vi "route.vi"() -> ()   [LabVIEW 2014]
uses:
  <vilib>/Utility/sysdir.llb/System Directory Type.ctl
  <vilib>/Utility/config.llb/Read Key (String).vi
  <vilib>/Utility/config.llb/Write Key (String).vi
  subVI/version.vi
  <vilib>/Utility/config.llb/Read Key (Path).vi
  <vilib>/Utility/config.llb/Write Key (Path).vi
  subVI/departure.vi
  subVI/Destination.vi
  <vilib>/Utility/file.llb/Write To Spreadsheet File (string).vi
  <vilib>/httpClient/LabVIEWHTTPClient.lvlib
  <vilib>/Utility/config.llb/NI_LVConfig.lvlib
panel:
  in  "ATC":bool
  out "활주로":string[](array[string])
  out "fms":string
  out "time/시간":dbl
  in  "도움말":bool
  in  "피드백":bool
  in  "저장 경로":path
  out "Distance":string="0"
  in  "찾기":bool
  in  "?":bool
  in  "?":bool
  out "x fmc 플랜":string
  out "FMS 플랜":string
  in  "Destination":string
  in  "departure":string
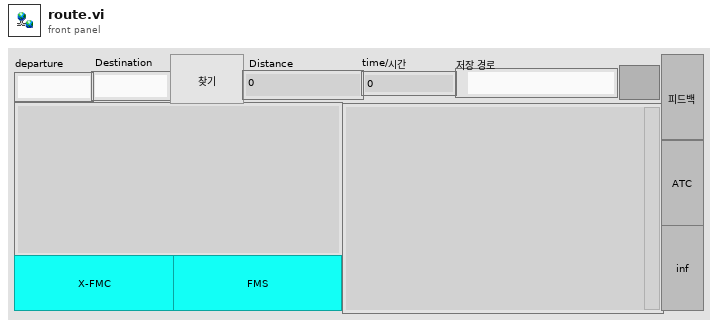
[diagram p1: front panel]
types:
  T1 = enum16{"open", "replace", "create", "open or create", "replace or create", "replace or create with confirmation"}
  T2 = typedef "NI_LVConfig.lvlib/Config Data RefNum.ctl" = refnum<k1>
  T3 = typedef "System Directory Type.ctl" = i32
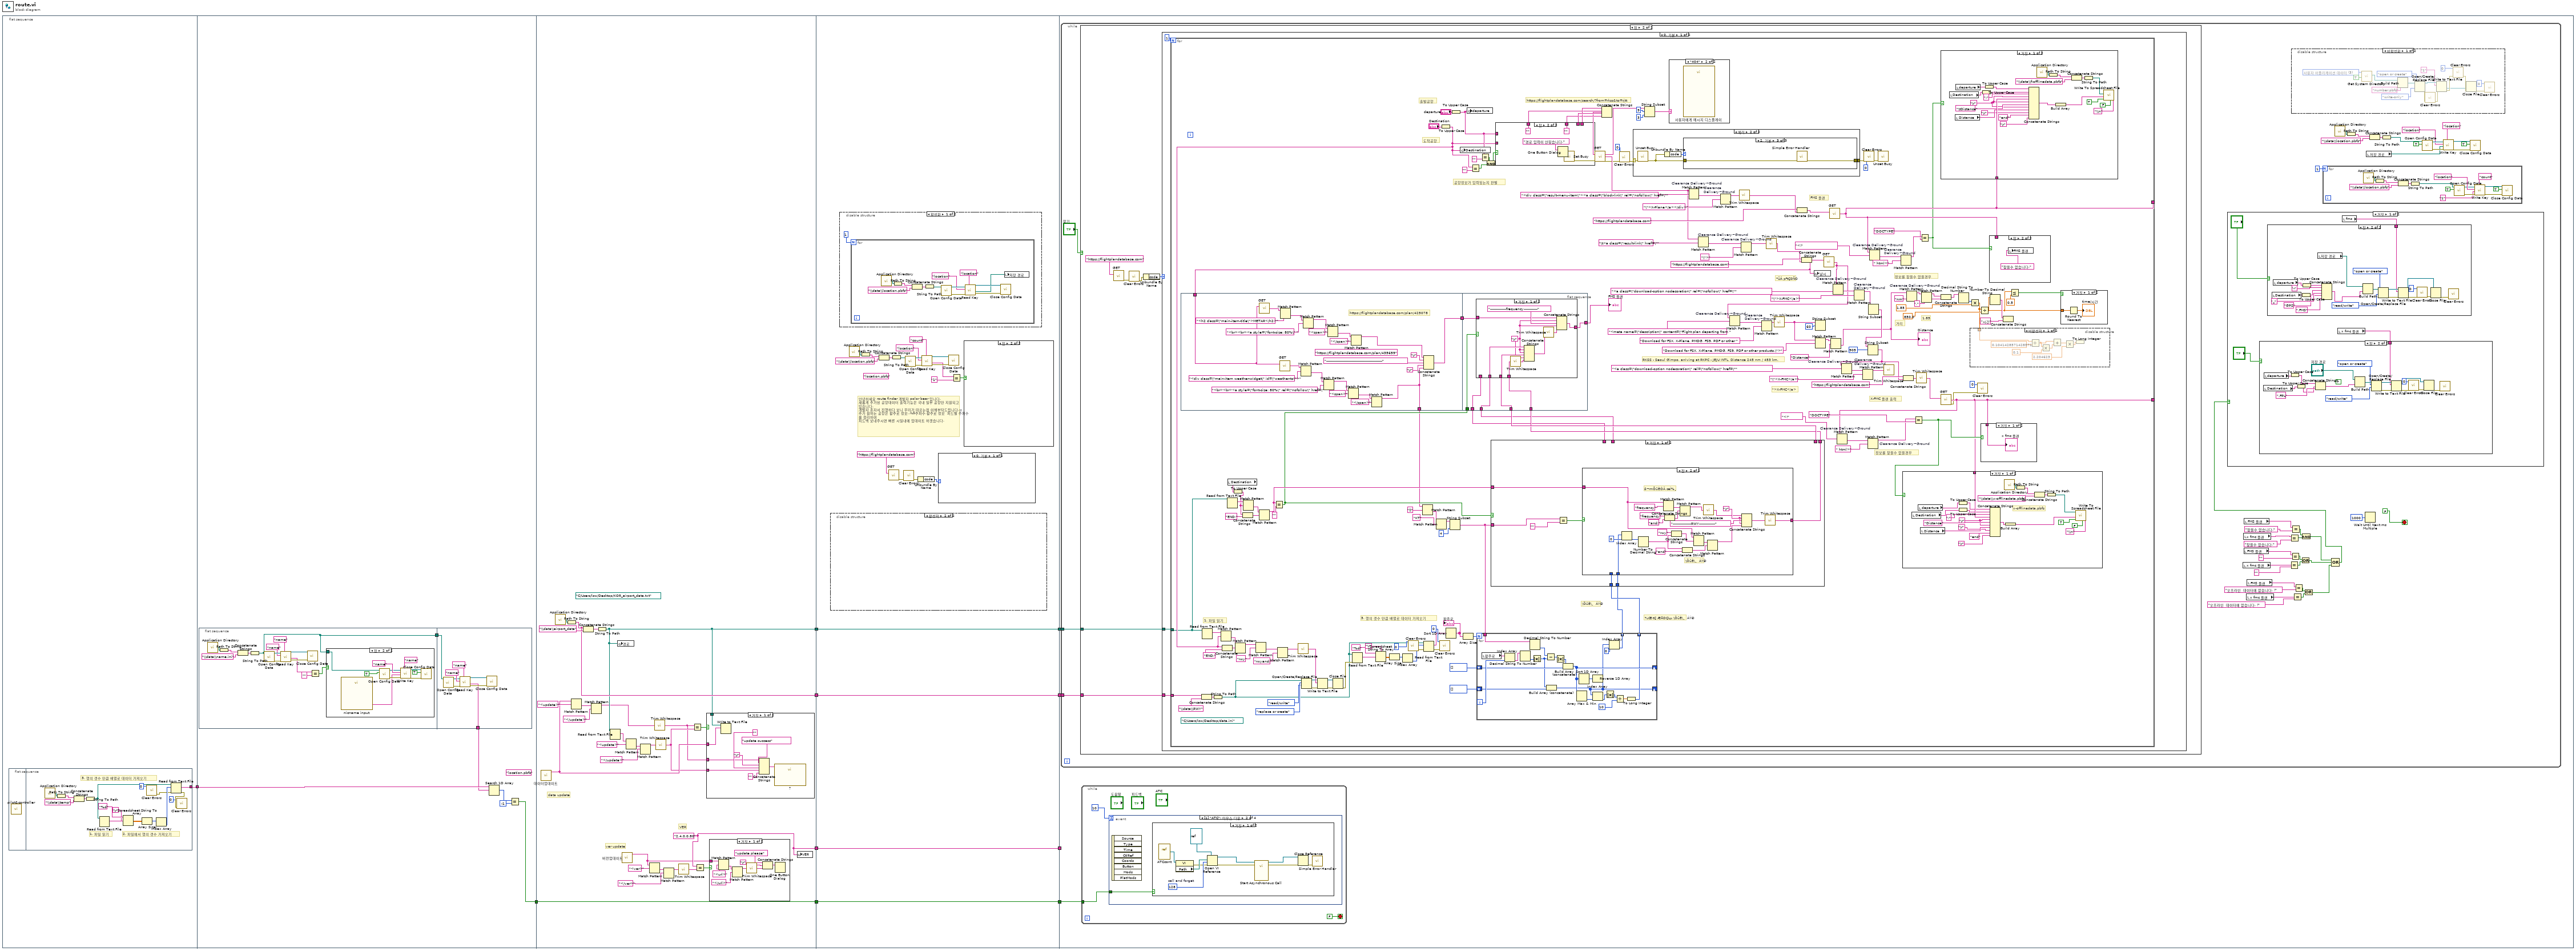
[diagram p0: block diagram]
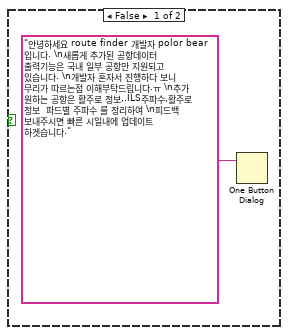
[diagram p5: hidden frame]
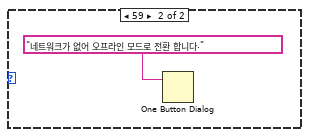
[diagram p6: hidden frame]
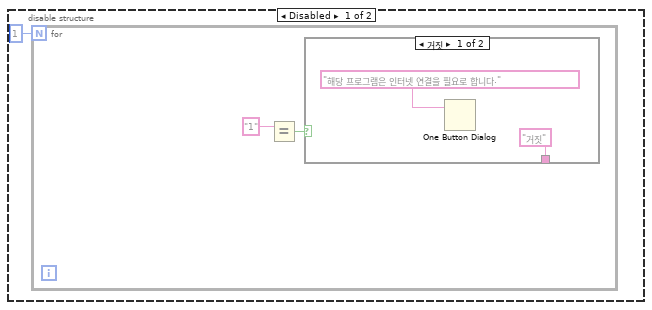
[diagram p7: hidden frame]
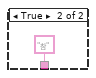
[diagram p8: hidden frame]
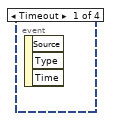
[diagram p10: hidden frame]
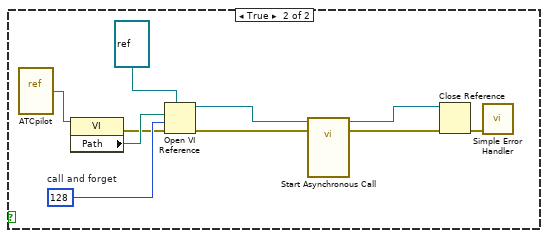
[diagram p11: hidden frame]
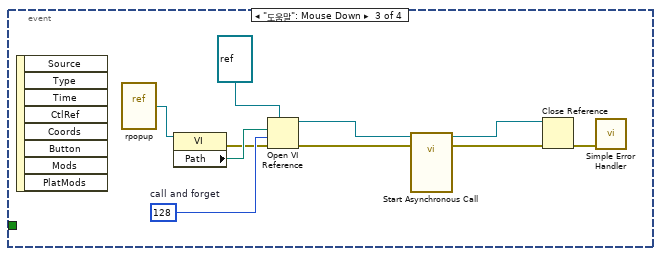
[diagram p12: hidden frame]
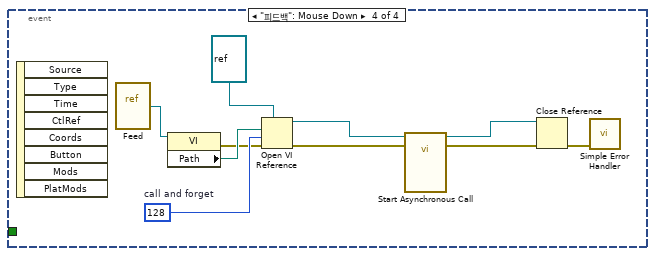
[diagram p13: hidden frame]
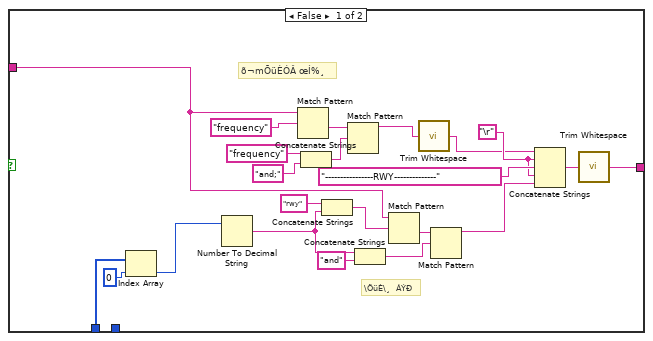
[diagram p15: hidden frame]
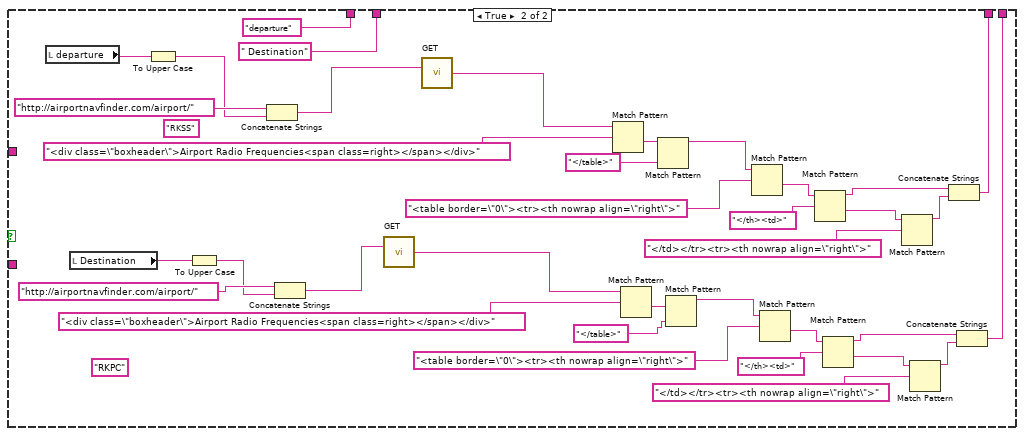
[diagram p16: hidden frame]
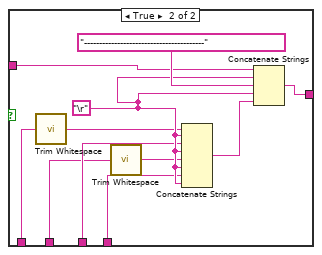
[diagram p17: hidden frame]
diagram:
  n1 = flat-sequence {
    tunnel: [w11] -> w4
    tunnel: w4 -> [w33]
    tunnel: [w31] -> w3
    tunnel: [w89] -> w8
    tunnel: [w90] -> w7
    tunnel: [w69] -> w6
    tunnel: w3 -> [w66]
    tunnel: [w66] -> w2
    tunnel: [w113] -> w10
    tunnel: [w114] -> w9
    tunnel: w8 -> [w113]
    tunnel: w7 -> [w114]
    tunnel: w6 -> [w112]
    tunnel: [w112] -> w5
    tunnel: w2 -> [w111]
    tunnel: [w111] -> w1
    tunnel: w10 -> [w156]
    tunnel: w9 -> [w155]
    tunnel: w5 -> [_]
    tunnel: w1 -> [w154]
    frame #0 {
      n2 = flat-sequence {
        tunnel: [w16] -> w11
        frame #0 {
          n3 = call "pilot&controller.vi"() -> ()  [unwired: 11 in, 1 out]
        }
        frame #1 {
          # "3. 행의 갯수 만큼 배열로 데이터 가져오기"
          # "2. 파일에서 행의 갯수 가져오기"
          # "1. 파일 읽기"
          n4 = call <vilib>:"Application Directory.vi"() -> ("Application Directory"=w20:path)
          n5 = Path To String(path=w20) -> (string=w19:string)
          n6 = Concatenate Strings(w19, "\\data\\temp" ("문자열")) -> (w18:string)
          n7 = String To Path(string=w18) -> (path=w17:path)
          n8 = Read from Text File(file (use dialog)=w17) -> (text=w23:string)  [unwired: 1 in, 5 out]
          n9 = Spreadsheet String To Array(delimiter (Tab)="\r", format string="%d", spreadsheet string=w23) -> (array=w25:dbl[][])  [unwired: 1 out]
          n10 = Array Size(array=w25) -> (size(s)=w24:i32[])
          n11 = call <vilib>:"Clear Errors.vi"("specific error code to clear (0: all)"=0) -> ("error out"=w15:errorcluster)  [unwired: 5 in, 1 out]
          n12 = Index Array(array=w24) -> (element=w22:i32)  [unwired: 1 in]
          n13 = Read from Text File(file (use dialog)=w17, count=w22, error in=w15) -> (text=w16:string[], error out=w13:errorcluster)  [unwired: 3 out]
          n14 = call <vilib>:"Clear Errors.vi"("error in (no error)"=w13, "specific error code to clear (0: all)"=0) -> ()  [unwired: 4 in, 2 out]
        }
      }
    }
    frame #1 {
      (unwired) "location.pbfs" ("문자열")
      n15 = flat-sequence {
        tunnel: [w34] -> w28
        tunnel: [w59] -> w30
        tunnel: w28 -> [w58]
        frame #0 {
          n16 = call <vilib>:"Application Directory.vi"() -> ("Application Directory"=w40:path)
          n17 = Path To String(path=w40) -> (string=w38:string)
          n18 = Concatenate Strings(w38, "\\data\\name.ini" ("문자열")) -> (w39:string)
          n19 = String To Path(string=w39) -> (path=w34:path)
          n20 = call <vilib>:"Open Config Data.vi"("configuration file path"=w34) -> ("error out"=w45:errorcluster, "refnum"=w46:T2)  [unwired: 8 in, 1 out]
          n21 = call-poly <vilib>:"Read Key.vi"("section"="name", "error in (no error)"=w45, "key"="name", "refnum"=w46) -> ("error out"=w44:errorcluster, "value"=w35:string, "refnum out"=w43:T2)  [unwired: 4 in, 1 out]
          n22 = call <vilib>:"Close Config Data.vi"("error in (no error)"=w44, "refnum"=w43) -> ()  [unwired: 8 in, 2 out]
          n23 = Equal?(x=w35, y="") -> (x = y?=w36:bool)
          n24 = case shown="참" w36 {
            tunnel: w34 -> [_ w48]
            frame False {
            }
            frame True {
              n25 = call "nicname input"() -> ("nicname"=w49:string)  [unwired: 17 in, 2 out]
              n26 = call <vilib>:"Open Config Data.vi"("create file if necessary (T)"=TRUE, "configuration file path"=w48) -> ("error out"=w51:errorcluster, "refnum"=w52:T2)  [unwired: 7 in, 1 out]
              n27 = call-poly <vilib>:"Write Key.vi"("section"="name", "error in (no error)"=w51, "value"=w49, "key"="name", "refnum"=w52) -> ("error out"=w54:errorcluster, "refnum out"=w53:T2)  [unwired: 4 in, 1 out]
              n28 = call <vilib>:"Close Config Data.vi"("error in (no error)"=w54, "write file if changed (T)"=TRUE, "refnum"=w53) -> ()  [unwired: 7 in, 2 out]
            }
          }
        }
        frame #1 {
          n29 = call <vilib>:"Open Config Data.vi"("configuration file path"=w58) -> ("error out"=w62:errorcluster, "refnum"=w61:T2)  [unwired: 8 in, 1 out]
          n30 = call-poly <vilib>:"Read Key.vi"("section"="name", "error in (no error)"=w62, "key"="name", "refnum"=w61) -> ("error out"=w63:errorcluster, "value"=w59:string, "refnum out"=w64:T2)  [unwired: 4 in, 1 out]
          n31 = call <vilib>:"Close Config Data.vi"("error in (no error)"=w63, "refnum"=w64) -> ()  [unwired: 8 in, 2 out]
        }
      }
      n32 = Search 1D Array(1D array=w33, element=w30) -> (index of element=w32:i32)  [unwired: 1 in]
      n33 = Equal?(x=w32, y=-1) -> (x = y?=w31:bool)
    }
    frame #2 {
      w69 = "2.4.0.0.80"
      (unwired) path "C:/Users/lsw/Desktop/KOR_airport_data.txt" ("File Path Control")
      # "ver update"
      # "data update"
      # "VER"
      n34 = call "데이터업데이트.vi"() -> ("data"=w78:string)  [unwired: 11 in]
      n35 = call <vilib>:"Application Directory.vi"() -> ("Application Directory"=w92:path)
      n36 = Path To String(path=w92) -> (string=w90:string)
      n37 = Match Pattern(string=w78, regular expression="<update>" ("정규식")) -> (after substring=w86:string)  [unwired: 1 in, 3 out]
      n38 = Concatenate Strings(w90, "\\data\\airport_data" ("문자열")) -> (w88:string)
      n39 = Match Pattern(string=w86, regular expression="</update>" ("정규식")) -> (before substring=w80:string)  [unwired: 1 in, 3 out]
      n40 = String To Path(string=w88) -> (path=w89:path)
      n41 = Read from Text File(file (use dialog)=w89) -> (text=w81:string)  [unwired: 3 in, 3 out]
      n42 = global write "airport경로.vi" "경로"(w89) -> ()
      n43 = call "버전업데이트.vi"() -> ("data"=w67:string)  [unwired: 11 in]
      n44 = Match Pattern(string=w81, regular expression="<update>" ("정규식")) -> (after substring=w83:string)  [unwired: 1 in, 3 out]
      n45 = Match Pattern(string=w83, regular expression="</update>" ("정규식")) -> (before substring=w79:string)  [unwired: 1 in, 3 out]
      n46 = Match Pattern(string=w67, regular expression="<ver>" ("정규식")) -> (after substring=w74:string)  [unwired: 1 in, 3 out]
      n47 = call <vilib>:"Trim Whitespace.vi"("string"=w80) -> ("trimmed string"=w76:string)  [unwired: 1 in]
      n48 = call <vilib>:"Trim Whitespace.vi"("string"=w79) -> ("trimmed string"=w77:string)  [unwired: 1 in]
      n49 = Match Pattern(string=w74, regular expression="</ver>" ("정규식")) -> (before substring=w71:string)  [unwired: 1 in, 3 out]
      n50 = call <vilib>:"Trim Whitespace.vi"("string"=w71) -> ("trimmed string"=w70:string)  [unwired: 1 in]
      n51 = Equal?(x=w76, y=w77) -> (x = y?=w75:bool)
      n52 = Equal?(x=w69, y=w70) -> (x = y?=w68:bool)
      n53 = case shown="거짓" w75 {
        tunnel: w89 -> [w110 _]
        tunnel: w78 -> [w104 _]
        tunnel: w77 -> [w103 _]
        tunnel: w76 -> [w102 _]
        frame False {
          n54 = Write to Text File(file (use dialog)=w110, text=w104) -> ()  [unwired: 2 in, 3 out]
          n55 = Concatenate Strings(w102, "update success" ("문자열"), "\r", "", w103, "" ("문자열")) -> (w105:string)
          n56 = call "?"("Message"=w105) -> ()  [unwired: 9 in, 2 out]
        }
        frame True {
        }
      }
      n57 = case shown="거짓" w68 {
        tunnel: w67 -> [w93 _]
        frame False {
          n58 = Match Pattern(string=w93, regular expression="<url>" ("정규식")) -> (after substring=w101:string)  [unwired: 1 in, 3 out]
          n59 = Match Pattern(string=w101, regular expression="</url>" ("정규식")) -> (before substring=w99:string)  [unwired: 1 in, 3 out]
          n60 = call <vilib>:"Trim Whitespace.vi"("string"=w99) -> ("trimmed string"=w97:string)  [unwired: 1 in]
          n61 = Concatenate Strings("update please" ("문자열"), "\r", w97) -> (w95:string)
          n62 = One Button Dialog(message=w95) -> ()  [unwired: 1 in, 1 out]
        }
        frame True {
        }
      }
      n63 = global write "version.vi" "VER"(w69) -> ()
    }
    frame #3 {
      (unwired) "location.pbfs" ("문자열")
      # "안녕하세요 route finder 개발자 polor bear 입니다. \n새롭게 추가된 공항데이터 출력기능은 국내 일부 공항만 지원되고 있습니다. \n개발자 혼자서 진행하다 보니 무리가 따르는점 이해부탁드립니다.ㅠ \n추가 원하는 공항은 활주로 정보,.ILS주파수,활주로 정보  파드별 주파수 를 정리하여 \n피드백 보내주시면 빠른 시일내에 업데이트 하겟습니다."
      n64 = disable-structure shown="활성화" {
        frame Disabled {
          n65 = for {
            N: 1 -> [_]
            n66 = Equal?(x="1" ("y")) -> (x = y?=w137:bool)  [unwired: 1 in]
            n67 = case shown="거짓" w137 {
              tunnel: ["거짓" "참"] -> _
              frame False {
                n68 = One Button Dialog(message="해당 프로그램은 인터넷 연결을 필요로 합니다." ("메시지")) -> ()  [unwired: 1 in, 1 out]
              }
              frame True {
              }
            }
          }
        }
        frame Enabled {
        }
      }
      n69 = disable-structure shown="활성화" {
        frame Enabled {
          n70 = for {
            N: 1 -> [_]
            n71 = call <vilib>:"Application Directory.vi"() -> ("Application Directory"=w145:path)
            n72 = Path To String(path=w145) -> (string=w143:string)
            n73 = Concatenate Strings(w143, "\\data\\location.pbfs" ("문자열")) -> (w144:string)
            n74 = String To Path(string=w144) -> (path=w142:path)
            n75 = call <vilib>:"Open Config Data.vi"("configuration file path"=w142) -> ("error out"=w151:errorcluster, "refnum"=w150:T2)  [unwired: 8 in, 1 out]
            n76 = call-poly <vilib>:"Read Key.vi"("section"="location", "error in (no error)"=w151, "key"="location", "refnum"=w150) -> ("error out"=w152:errorcluster, "value"=w147:path, "refnum out"=w153:T2)  [unwired: 4 in, 1 out]
            n77 = call <vilib>:"Close Config Data.vi"("error in (no error)"=w152, "refnum"=w153) -> ()  [unwired: 8 in, 2 out]
            n78 = local write "저장 경로"(w147) -> ()
          }
        }
        frame Disabled {
        }
      }
      n79 = call <vilib>:"Application Directory.vi"() -> ("Application Directory"=w118:path)
      n80 = Path To String(path=w118) -> (string=w116:string)
      n81 = Concatenate Strings(w116, "\\data\\location.pbfs" ("문자열")) -> (w117:string)
      n82 = call <vilib>:"GET.vi"("url"="https://flightplandatabase.com") -> ("error out"=w132:errorcluster)  [unwired: 11 in, 3 out]
      n83 = String To Path(string=w117) -> (path=w115:path)
      n84 = call <vilib>:"Clear Errors.vi"("error in (no error)"=w132) -> ("error out"=w130:errorcluster)  [unwired: 5 in, 1 out]
      n85 = call <vilib>:"Open Config Data.vi"("configuration file path"=w115) -> ("error out"=w126:errorcluster, "refnum"=w127:T2)  [unwired: 8 in, 1 out]
      n86 = Unbundle By Name(w130) -> ("code"=w129:i32)
      n87 = call-poly <vilib>:"Read Key.vi"("section"="count", "error in (no error)"=w126, "key"="location", "refnum"=w127) -> ("error out"=w125:errorcluster, "value"=w120:string, "refnum out"=w124:T2)  [unwired: 4 in, 1 out]
      n88 = case shown="0, 기본" w129 {
        frame 0, Default {
        }
        frame 59 {
          n89 = One Button Dialog(message="네트워크가 없어 오프라인 모드로 전환 합니다." ("메시지")) -> ()  [unwired: 1 in, 1 out]
        }
      }
      n90 = call <vilib>:"Close Config Data.vi"("error in (no error)"=w125, "refnum"=w124) -> ()  [unwired: 8 in, 2 out]
      n91 = Equal?(x=w120, y="1") -> (x = y?=w122:bool)
      n92 = case shown="참" w122 {
        frame False {
          n93 = One Button Dialog(message="안녕하세요 route finder 개발자 polor bear 입니다. \n새롭게 추가된 공항데이터 출력기능은 국내 일부 공항만 지원되고 있습니다. \n개발자 혼자서 진행하다 보니 무리가 따르는점 이해부탁드립니다.ㅠ \n추가 원하는 공항은 활주로 정보,.ILS주파수,활주로 정보  파드별 주파수 를 정리하여 \n피드백 보내주시면 빠른 시일내에 업데이트 하겟습니다." ("메시지")) -> ()  [unwired: 1 in, 1 out]
        }
        frame True {
        }
      }
    }
    frame #4 {
      n94 = while {
        tunnel: w156 -> [w209]
        tunnel: w155 -> [w208]
        stop <- FALSE stop-if-true
        n95 = case shown="참" "찾기" {
          tunnel: w209 -> [_ w258]
          tunnel: w208 -> [_ w257]
          frame False {
          }
          frame True {
            n96 = call <vilib>:"GET.vi"("url"="https://flightplandatabase.com") -> ("error out"=w262:errorcluster)  [unwired: 11 in, 3 out]
            n97 = call <vilib>:"Clear Errors.vi"("error in (no error)"=w262) -> ("error out"=w260:errorcluster)  [unwired: 5 in, 1 out]
            n98 = Unbundle By Name(w260) -> ("code"=w259:i32)
            n99 = case shown="0, 기본" w259 {
              tunnel: w258 -> [w265 _]
              tunnel: w257 -> [w264 _]
              frame 0, Default {
                n100 = for {
                  N: 1 -> [_]
                  tunnel: [w336] -> _
                  tunnel: [w341] -> _
                  tunnel: w265 -> [w303]
                  tunnel: w264 -> [w313]
                  (unwired) path "C:/Users/lsw/Desktop/data.ini" ("File Path Control")
                  # "¼Œ·tÇ ÆÅDÇLµ \\ÖüÈ\\¸  ÁÝÐ"
                  # "\\ÖüÈ\\¸  ÁÝÐ"
                  # "1. 파일 읽기"
                  # "3. 행의 갯수 만큼 배열로 데이터 가져오기"
                  # "°ÜÂ p³tÇ0ÑO"
                  # "1.85"
                  # "RKSS - Seoul Gimpo, arriving at RKPC - JEJU INTL. Distance 245 nm / 453 km."
                  # "\">X-FMC</a>"
                  # "https://flightplandatabase.com/search/?from=rkss&to=rjtt"
                  # "FMS 플랜"
                  # "거리"
                  # "X-FMC 플랜 출력"
                  # "정보를 찾을수 없을경우"
                  # "정보를 찾을수 없을경우"
                  # "공항정보가 입력됫는지 판별"
                  # "도착공항"
                  # "출발공항"
                  n101 = flat-sequence {
                    tunnel: w324 -> [w534]
                    tunnel: [w533] -> w319
                    tunnel: [w532] -> w302
                    tunnel: w321 -> [w561]
                    tunnel: w320 -> [w559]
                    tunnel: w319 -> [w560]
                    tunnel: w317 -> [w558]
                    tunnel: w316 -> [w555]
                    tunnel: [w557] -> w314
                    tunnel: w315 -> [w556]
                    frame #0 {
                      (unwired) "https://flightplandatabase.com/plan/435659"
                      # "https://flightplandatabase.com/plan/425078"
                      n102 = call <vilib>:"GET.vi"("url"=w534) -> ("body"=w554:string)  [unwired: 11 in, 3 out]
                      n103 = call <vilib>:"GET.vi"("url"=w534) -> ("body"=w539:string)  [unwired: 11 in, 3 out]
                      n104 = Match Pattern(string=w554, regular expression="<h2 class=\"main-item-title\">METAR</h2>" ("정규식")) -> (after substring=w552:string)  [unwired: 1 in, 3 out]
                      n105 = Match Pattern(string=w539, regular expression="<div class=\"main-item weather-widget\" id=\"weather-to\">" ("정규식")) -> (after substring=w541:string)  [unwired: 1 in, 3 out]
                      n106 = Match Pattern(string=w552, regular expression="<br><br><a style=\"font-size: 80%\" " ("정규식")) -> (before substring=w550:string)  [unwired: 1 in, 3 out]
                      n107 = Match Pattern(string=w541, regular expression="<br><br><a style=\"font-size: 80%\" rel=\"nofollow\" href=\"" ("정규식")) -> (before substring=w543:string)  [unwired: 1 in, 3 out]
                      n108 = Match Pattern(string=w550, regular expression="<span>" ("정규식")) -> (after substring=w548:string)  [unwired: 1 in, 3 out]
                      n109 = Match Pattern(string=w543, regular expression="<span>" ("정규식")) -> (after substring=w545:string)  [unwired: 1 in, 3 out]
                      n110 = Match Pattern(string=w548, regular expression="</span>" ("정규식")) -> (before substring=w536:string)  [unwired: 1 in, 3 out]
                      n111 = Match Pattern(string=w545, regular expression="</span>" ("정규식")) -> (before substring=w532:string)  [unwired: 1 in, 3 out]
                      n112 = Concatenate Strings(w536, "\r", "-------------------------------------------------" ("문자열"), "\r", w532) -> (w533:string)
                    }
                    frame #1 {
                      n113 = case shown="거짓" w556 {
                        tunnel: w561 -> [w569 w579]
                        tunnel: w560 -> [w570 w578]
                        tunnel: w559 -> [w562 w577]
                        tunnel: w558 -> [_ w575]
                        tunnel: w555 -> [w565 w573]
                        tunnel: [w568 w572] -> w557
                        frame False {
                          w564 = "\r"
                          n114 = call <vilib>:"Trim Whitespace.vi"("string"=w562) -> ("trimmed string"=w563:string)  [unwired: 1 in]
                          n115 = Concatenate Strings(w565, w564, w564, w569, w564, w563) -> (w566:string)
                          n116 = call <vilib>:"Trim Whitespace.vi"("string"=w566) -> ("trimmed string"=w567:string)  [unwired: 1 in]
                          n117 = Concatenate Strings(w570, w564, "--------------frequency------------" ("문자열"), w564, w567) -> (w568:string)
                        }
                        frame True {
                          w580 = "\r"
                          n118 = call <vilib>:"Trim Whitespace.vi"("string"=w575) -> ("trimmed string"=w576:string)  [unwired: 1 in]
                          n119 = call <vilib>:"Trim Whitespace.vi"("string"=w573) -> ("trimmed string"=w574:string)  [unwired: 1 in]
                          n120 = Concatenate Strings(w576, w580, w579, w580, w574, w580, w577, w580) -> (w581:string)
                          n121 = Concatenate Strings(w578, w580, "----------------------------------------" ("문자열"), w580, w581) -> (w572:string)
                        }
                      }
                    }
                  }
                  n122 = Concatenate Strings(w313, "\\data\\RWY" ("문자열")) -> (w271:string)
                  n123 = Read from Text File(file (use dialog)=w303) -> (text=w284:string)  [unwired: 1 in, 5 out]
                  n124 = String To Path(string=w271) -> (path=w266:path)
                  n125 = Read from Text File(file (use dialog)=w303) -> (text=w310:string)  [unwired: 1 in, 5 out]
                  n126 = local read "Destination"() -> (w304:string)
                  n127 = To Upper Case(1:w304) -> (0:w305:string)
                  n128 = Concatenate Strings(w305, "END;" ("정규식")) -> (w308:string)
                  n129 = Match Pattern(string=w310, regular expression=w305) -> (after substring=w306:string)  [unwired: 1 in, 3 out]
                  n130 = Match Pattern(string=w306, regular expression=w308) -> (before substring=w318:string)  [unwired: 1 in, 3 out]
                  n131 = Equal?(x=w318, y="") -> (x = y?=w315:bool)
                  n132 = Open/Create/Replace File(file path (use dialog)=w266, operation (0:open)=T1."replace or create" ("동작(0:open)"), access (0:read/write)=enum16{"read/write", "read-only", "write-only"}."read/write" ("접근(0:읽기/쓰기)")) -> (refnum out=w274:refnum<file>, error out=w277:errorcluster)  [unwired: 3 in, 1 out]
                  n133 = call <vilib>:"Clear Errors.vi"("specific error code to clear (0: all)"=0) -> ("error out"=w292:errorcluster)  [unwired: 5 in, 1 out]
                  n134 = Match Pattern(string=w302, regular expression="Z" ("정규식")) -> (after substring=w326:string)  [unwired: 1 in, 3 out]
                  n135 = Match Pattern(string=w326, regular expression="KT" ("정규식")) -> (before substring=w323:string)  [unwired: 1 in, 3 out]
                  n136 = To Upper Case(1:"Destination") -> (0:w328:string)
                  n137 = Match Pattern(string=w284, regular expression=w328) -> (after substring=w285:string)  [unwired: 1 in, 3 out]
                  n138 = Concatenate Strings(w328, "END;" ("정규식")) -> (w282:string)
                  n139 = Match Pattern(string=w285, regular expression=w282) -> (before substring=w283:string)  [unwired: 1 in, 3 out]
                  n140 = Match Pattern(string=w283, regular expression="rwy" ("문자열")) -> (after substring=w280:string)  [unwired: 1 in, 3 out]
                  n141 = Match Pattern(string=w280, regular expression="rwyand;" ("정규식")) -> (before substring=w279:string)  [unwired: 1 in, 3 out]
                  n142 = call <vilib>:"Trim Whitespace.vi"("string"=w279) -> ("trimmed string"=w278:string)  [unwired: 1 in]
                  n143 = Write to Text File(file (use dialog)=w274, text=w278, error in=w277) -> (refnum out=w275:refnum<file>, error out=w276:errorcluster)  [unwired: 1 in, 1 out]
                  n144 = Close File(refnum=w275, error in=w276) -> (error out=w312:errorcluster)  [unwired: 1 out]
                  n145 = Read from Text File(file (use dialog)=w266, error in=w312) -> (text=w297:string)  [unwired: 5 out]
                  n146 = Spreadsheet String To Array(delimiter (Tab)="\r", format string="%d", spreadsheet string=w297) -> (array=w295:dbl[][])  [unwired: 1 out]
                  n147 = Array Size(array=w295) -> (size(s)=w296:i32[])
                  n148 = Index Array(array=w296) -> (element=w298:i32)  [unwired: 1 in]
                  n149 = Read from Text File(file (use dialog)=w266, count=w298, error in=w292) -> (text=w288:string[], error out=w290:errorcluster)  [unwired: 3 out]
                  n150 = call <vilib>:"Clear Errors.vi"("error in (no error)"=w290, "specific error code to clear (0: all)"=0) -> ()  [unwired: 4 in, 2 out]
                  n151 = Sort 1D Array(array=w288) -> (sorted array=w311:string[])
                  "활주로" <- w311
                  n152 = String Subset(string=w323, length (rest)=4 ("길이(나머지)")) -> (substring=w268:string)  [unwired: 1 in]
                  n153 = To Upper Case(1:"departure") -> (0:w330:string)
                  n154 = global write "Destination.vi" "Destination"(w328) -> ()
                  n155 = Array Size(array=w311) -> (size(s)=w300:i32)
                  n156 = global write "departure.vi" "departure"(w330) -> ()
                  n157 = Equal?(x=w328, y="") -> (x = y?=w367:bool)
                  n158 = for {
                    N: w300 -> [_]
                    shift-right: [w439] -> _
                    shift-left: i32[] [] -> [w443]
                    shift-right: [w425] -> _
                    shift-left: i32[] [] -> [w437]
                    tunnel: w268 -> [w429]
                    tunnel: [w426] -> w269 mode=indexing
                    tunnel: [w423] -> w267 mode=indexing
                    i -> [w444]
                    n159 = local read "활주로"() -> (w442:string[])
                    n160 = Index Array(array=w442, index=w444) -> (element=w441:string)
                    n161 = Decimal String To Number(string=w441) -> (number=w433:i32)  [unwired: 2 in, 1 out]
                    n162 = Decimal String To Number(string=w429) -> (number=w428:i32)  [unwired: 2 in, 1 out]
                    n163 = Absolute Value(x=w433) -> (abs(x)=w427:i32)
                    n164 = Subtract(x=w428, y=w427) -> (x-y=w432:i32)
                    n165 = Build Array (concatenate)(w427, w437) -> (w425:i32[])
                    n166 = Absolute Value(x=w432) -> (abs(x)=w431:i32)
                    n167 = Build Array (concatenate)(w431, w443) -> (w439:i32[])
                    n168 = Array Max & Min(array=w439) -> (min index (indices)=w438:i32)  [unwired: 3 out]
                    n169 = Sort 1D Array(array=w439) -> (sorted array=w440:i32[])
                    n170 = Reverse 1D Array(array=w440) -> ()  [unwired: 1 out]
                    n171 = Index Array(array=w425, index=w438) -> (element=w434:i32)
                    n172 = Absolute Value(x=w434) -> (abs(x)=w435:i32)
                    n173 = Index Array(array=w425, index=0 ("인덱스")) -> (element=w423:i32)
                    n174 = Divide(x=w435, y=10) -> (x/y=w430:dbl)
                    n175 = To Long Integer(number=w430) -> (32bit integer=w426:i32)
                  }
                  n176 = Equal?(x=w330, y="") -> (x = y?=w366:bool)
                  n177 = And(x=w366, y=w367) -> (x .and. y?=w368:bool)
                  n178 = case shown="거짓" w315 {
                    tunnel: [_ w503] -> w321
                    tunnel: [w450 w502] -> w320
                    tunnel: w318 -> [w451 _]
                    tunnel: [_ "departure"] -> w317
                    tunnel: [_ " Destination"] -> w316
                    tunnel: w269 -> [w449 _]
                    tunnel: w268 -> [w447 _]
                    tunnel: w267 -> [w445 _]
                    frame False {
                      n179 = Equal?(x=w447, y="") -> (x = y?=w448:bool)
                      n180 = case shown="참" w448 {
                        tunnel: w451 -> [w465 w477]
                        tunnel: [w457 w478] -> w450
                        tunnel: w449 -> [w454 _]
                        tunnel: w445 -> [_ w475]
                        frame False {
                          w460 = "\r"
                          # "õ¬mÕüÈÓÂ œÍ%¸"
                          # "\\ÖüÈ\\¸  ÁÝÐ"
                          n181 = Index Array(array=w454, index=0 ("인덱스")) -> (element=w452:i32)
                          n182 = Number To Decimal String(number=w452) -> (decimal integer string=w466:string)  [unwired: 1 in]
                          n183 = Match Pattern(string=w465, regular expression="frequency") -> (after substring=w470:string)  [unwired: 1 in, 3 out]
                          n184 = Concatenate Strings("frequency", "and;") -> (w469:string)
                          n185 = Concatenate Strings("rwy", w466) -> (w464:string)
                          n186 = Match Pattern(string=w470, regular expression=w469) -> (before substring=w456:string)  [unwired: 1 in, 3 out]
                          n187 = Concatenate Strings(w466, "and") -> (w462:string)
                          n188 = Match Pattern(string=w465, regular expression=w464) -> (after substring=w463:string)  [unwired: 1 in, 3 out]
                          n189 = call <vilib>:"Trim Whitespace.vi"("string"=w456) -> ("trimmed string"=w455:string)  [unwired: 1 in]
                          n190 = Match Pattern(string=w463, regular expression=w462) -> (before substring=w459:string)  [unwired: 1 in, 3 out]
                          n191 = Concatenate Strings(w455, w460, "----------------RWY--------------", w460, w459) -> (w458:string)
                          n192 = call <vilib>:"Trim Whitespace.vi"("string"=w458) -> ("trimmed string"=w457:string)  [unwired: 1 in]
                        }
                        frame True {
                          w483 = "\r"
                          # "õ¬mÕüÈÓÂ œÍ%¸"
                          # "\\ÖüÈ\\¸  ÁÝÐ"
                          n193 = Index Array(array=w475, index=0 ("인덱스")) -> (element=w474:i32)
                          n194 = Number To Decimal String(number=w474) -> (decimal integer string=w488:string)  [unwired: 1 in]
                          n195 = Match Pattern(string=w477, regular expression="frequency") -> (after substring=w492:string)  [unwired: 1 in, 3 out]
                          n196 = Concatenate Strings("frequency", "and;") -> (w491:string)
                          n197 = Concatenate Strings("rwy", w488) -> (w487:string)
                          n198 = Match Pattern(string=w492, regular expression=w491) -> (before substring=w480:string)  [unwired: 1 in, 3 out]
                          n199 = Concatenate Strings(w488, "and") -> (w485:string)
                          n200 = Match Pattern(string=w477, regular expression=w487) -> (after substring=w486:string)  [unwired: 1 in, 3 out]
                          n201 = call <vilib>:"Trim Whitespace.vi"("string"=w480) -> ("trimmed string"=w479:string)  [unwired: 1 in]
                          n202 = Match Pattern(string=w486, regular expression=w485) -> (before substring=w482:string)  [unwired: 1 in, 3 out]
                          n203 = Concatenate Strings(w479, w483, "----------------RWY--------------", w483, w482) -> (w481:string)
                          n204 = call <vilib>:"Trim Whitespace.vi"("string"=w481) -> ("trimmed string"=w478:string)  [unwired: 1 in]
                        }
                      }
                    }
                    frame True {
                      (unwired) "RKPC" ("문자열")
                      (unwired) "RKSS" ("문자열")
                      n205 = local read "departure"() -> (w499:string)
                      n206 = local read "Destination"() -> (w497:string)
                      n207 = To Upper Case(1:w499) -> (0:w498:string)
                      n208 = To Upper Case(1:w497) -> (0:w496:string)
                      n209 = Concatenate Strings("http://airportnavfinder.com/airport/", w498) -> (w531:string)
                      n210 = Concatenate Strings("http://airportnavfinder.com/airport/", w496) -> (w505:string)
                      n211 = call <vilib>:"GET.vi"("url"=w505) -> ("body"=w507:string)  [unwired: 11 in, 3 out]
                      n212 = call <vilib>:"GET.vi"("url"=w531) -> ("body"=w529:string)  [unwired: 11 in, 3 out]
                      n213 = Match Pattern(string=w529, regular expression="<div class=\"boxheader\">Airport Radio Frequencies<span class=right></span></div>" ("정규식")) -> (after substring=w527:string)  [unwired: 1 in, 3 out]
                      n214 = Match Pattern(string=w507, regular expression="<div class=\"boxheader\">Airport Radio Frequencies<span class=right></span></div>" ("정규식")) -> (after substring=w509:string)  [unwired: 1 in, 3 out]
                      n215 = Match Pattern(string=w527, regular expression="</table>" ("정규식")) -> (before substring=w525:string)  [unwired: 1 in, 3 out]
                      n216 = Match Pattern(string=w509, regular expression="</table>" ("정규식")) -> (before substring=w504:string)  [unwired: 1 in, 3 out]
                      n217 = Match Pattern(string=w525, regular expression="<table border=\"0\"><tr><th nowrap align=\"right\">" ("정규식")) -> (after substring=w523:string)  [unwired: 1 in, 3 out]
                      n218 = Match Pattern(string=w504, regular expression="<table border=\"0\"><tr><th nowrap align=\"right\">" ("정규식")) -> (after substring=w512:string)  [unwired: 1 in, 3 out]
                      n219 = Match Pattern(string=w523, regular expression="</th><td>" ("정규식")) -> (before substring=w519:string, after substring=w521:string)  [unwired: 1 in, 2 out]
                      n220 = Match Pattern(string=w512, regular expression="</th><td>" ("정규식")) -> (before substring=w516:string, after substring=w514:string)  [unwired: 1 in, 2 out]
                      n221 = Match Pattern(string=w521, regular expression="</td></tr><tr><th nowrap align=\"right\">" ("정규식")) -> (before substring=w518:string)  [unwired: 1 in, 3 out]
                      n222 = Match Pattern(string=w514, regular expression="</td></tr><tr><th nowrap align=\"right\">" ("정규식")) -> (before substring=w517:string)  [unwired: 1 in, 3 out]
                      n223 = Concatenate Strings(w519, w518) -> (w503:string)
                      n224 = Concatenate Strings(w516, w517) -> (w502:string)
                    }
                  }
                  n225 = case shown="참" w368 {
                    tunnel: ["&to=" ("문자열") _] -> w358
                    tunnel: ["https://flightplandatabase.com/search/?from=" ("문자열") _] -> w357
                    tunnel: w328 -> [w639 _]
                    tunnel: [w639 "" ("Destination")] -> w356
                    tunnel: [w638 "" ("departure")] -> w355
                    tunnel: w330 -> [w638 _]
                    frame False {
                    }
                    frame True {
                      n226 = One Button Dialog(message="경로 입력이 안됫습니다." ("메시지")) -> ()  [unwired: 1 in, 1 out]
                    }
                  }
                  n227 = call <vilib>:"Set Busy.vi"() -> ("error out"=w418:errorcluster)  [unwired: 10 in, 1 out]
                  n228 = Concatenate Strings(w357, w355, w358, w356) -> (w339:string)
                  n229 = call <vilib>:"GET.vi"("url"=w339, "error in (no error)"=w418) -> ("headers"=w422:string, "body"=w392:string, "error out"=w377:errorcluster)  [unwired: 10 in, 1 out]
                  n230 = call <vilib>:"Clear Errors.vi"("error in (no error)"=w377, "specific error code to clear (0: all)"=0) -> ("error out"=w378:errorcluster)  [unwired: 4 in, 1 out]
                  n231 = case shown="에러" w378 {
                    selector: w378 -> [w649 w652]
                    tunnel: [w649 w650] -> w374
                    frame No Error {
                    }
                    frame Error {
                      n232 = call <vilib>:"Unset Busy.vi"("error in (no error)"=w652) -> ("error out"=w651:errorcluster)  [unwired: 10 in]
                      n233 = Unbundle By Name(w651) -> ("code"=w653:i32)
                      n234 = case shown="2, 기본" w653 {
                        tunnel: w651 -> [w654 w659 w661]
                        tunnel: [w654 w659 w660] -> w650
                        frame 59 {
                          n235 = One Button Dialog(message="에러가 발생하였습니다. 종료하려면 확인 버튼을 누르세요" ("메시지")) -> (true=w655:bool)  [unwired: 1 in]
                          n236 = Stop(stop? (T)=w655) -> ()
                        }
                        frame 1 {
                          n237 = One Button Dialog(message="루트를 입력하여 주세요. 종료하려면 확인 버튼을 눌러 주세요" ("메시지")) -> (true=w657:bool)  [unwired: 1 in]
                          n238 = Stop(stop? (T)=w657) -> ()
                        }
                        frame 2, Default {
                          n239 = call <vilib>:"Simple Error Handler.vi"("error in (no error)"=w661) -> ("error out"=w660:errorcluster)  [unwired: 4 in, 4 out]
                        }
                      }
                    }
                  }
                  n240 = String Subset(string=w422, offset (0)=9 ("오프셋(0)"), length (rest)=3 ("길이(나머지)")) -> (substring=w419:string)
                  n241 = case shown="\"404\"" w419 {
                    frame "거짓", Default {
                    }
                    frame "404" {
                      n242 = call "사용자에게 메시지 디스플레이"() -> ()  [unwired: 10 in, 2 out]
                    }
                  }
                  n243 = Match Pattern "Clearance Delivery~Ground"(string=w392, regular expression="<div class=\"result-menu-item\"><a class=\"block-link\" rel=\"nofollow\" href=\"" ("정규식")) -> (after substring=w416:string)  [unwired: 1 in, 3 out]
                  n244 = Match Pattern "Clearance Delivery~Ground"(string=w392, regular expression="\t<a class=\"result-link\" href=\"" ("정규식")) -> (after substring=w410:string)  [unwired: 1 in, 3 out]
                  n245 = Match Pattern "Clearance Delivery~Ground"(string=w416, regular expression="\">X-Plane</a></div>" ("정규식")) -> (before substring=w414:string)  [unwired: 1 in, 3 out]
                  n246 = call <vilib>:"Trim Whitespace.vi"("string"=w414) -> ("trimmed string"=w411:string)  [unwired: 1 in]
                  n247 = Match Pattern "Clearance Delivery~Ground"(string=w410, regular expression="\">" ("정규식")) -> (before substring=w407:string)  [unwired: 1 in, 3 out]
                  n248 = call <vilib>:"Trim Whitespace.vi"("string"=w407) -> ("trimmed string"=w405:string)  [unwired: 1 in]
                  n249 = Concatenate Strings("https://flightplandatabase.com" ("url"), w411) -> (w412:string)
                  n250 = Concatenate Strings("https://flightplandatabase.com" ("url"), w405) -> (w324:string)
                  n251 = global write "날시.vi" "날시"(w324) -> ()
                  n252 = call <vilib>:"GET.vi"("url"=w324) -> ("body"=w338:string)  [unwired: 11 in, 3 out]
                  n253 = Match Pattern "Clearance Delivery~Ground"(string=w338, regular expression="<meta name=\"description\" content=\"Flight plan departing from " ("정규식")) -> (after substring=w393:string)  [unwired: 1 in, 3 out]
                  n254 = Match Pattern "Clearance Delivery~Ground"(string=w393, regular expression="Download for FSX, X-Plane, PMDG, FS9, PDF or other " ("정규식")) -> (before substring=w395:string)  [unwired: 1 in, 3 out]
                  n255 = call <vilib>:"Trim Whitespace.vi"("string"=w395) -> ("trimmed string"=w363:string)  [unwired: 1 in]
                  n256 = String Subset(string=w363, offset (0)=60 ("오프셋(0)")) -> ()  [unwired: 1 in, 1 out]
                  n257 = Match Pattern(string=w363, regular expression="Download for FSX, X-Plane, PMDG, FS9, PDF or other products.\">" ("정규식")) -> (before substring=w361:string)  [unwired: 1 in, 3 out]
                  n258 = call <vilib>:"GET.vi"("url"=w412) -> ("body"=w341:string)  [unwired: 11 in, 3 out]
                  n259 = Match Pattern(string=w361, regular expression="Distance" ("정규식")) -> (after substring=w359:string)  [unwired: 1 in, 3 out]
                  "Distance" <- w359
                  n260 = Match Pattern "Clearance Delivery~Ground"(string=w338, regular expression="<a class=\"download-option nodecoration\" rel=\"nofollow\" href=\"" ("정규식")) -> (after substring=w402:string)  [unwired: 1 in, 3 out]
                  n261 = Match Pattern "Clearance Delivery~Ground"(string=w402, regular expression="\">X-FMC</a>" ("정규식")) -> (before substring=w401:string)  [unwired: 1 in, 3 out]
                  n262 = call <vilib>:"Clear Errors.vi"("error in (no error)"=w374, "specific error code to clear (0: all)"=0) -> ("error out"=w375:errorcluster)  [unwired: 4 in, 1 out]
                  n263 = String Subset(string=w401) -> (substring=w364:string)  [unwired: 2 in]
                  n264 = String Subset(string=w364, offset (0)=905 ("오프셋(0)")) -> (substring=w332:string)  [unwired: 1 in]
                  n265 = Match Pattern "Clearance Delivery~Ground"(string=w332, regular expression="<a class=\"download-option nodecoration\" rel=\"nofollow\" href=\"" ("정규식")) -> (after substring=w398:string)  [unwired: 1 in, 3 out]
                  n266 = Match Pattern "Clearance Delivery~Ground"(string=w398, regular expression="\">X-FMC</a>" ("정규식")) -> (before substring=w333:string)  [unwired: 1 in, 3 out]
                  n267 = Match Pattern "Clearance Delivery~Ground"(string=w341, regular expression="<!" ("문자열")) -> (after substring=w388:string)  [unwired: 1 in, 3 out]
                  n268 = call <vilib>:"Unset Busy.vi"("error in (no error)"=w375) -> ()  [unwired: 10 in, 1 out]
                  n269 = call <vilib>:"Trim Whitespace.vi"("string"=w333) -> ()  [unwired: 1 in, 1 out]
                  n270 = Match Pattern "Clearance Delivery~Ground"(string=w388, regular expression=" html>" ("정규식")) -> (before substring=w387:string)  [unwired: 1 in, 3 out]
                  n271 = Concatenate Strings("https://flightplandatabase.com" ("url"), w332) -> (w396:string)
                  n272 = Match Pattern "Clearance Delivery~Ground"(string=w359, regular expression="nm" ("정규식")) -> (before substring=w351:string)  [unwired: 1 in, 3 out]
                  n273 = call <vilib>:"Trim Whitespace.vi"("string"=w396) -> ("trimmed string"=w337:string)  [unwired: 1 in]
                  n274 = Equal?(x=w387, y="DOCTYPE") -> (x = y?=w340:bool)
                  n275 = Match Pattern(string=w351, regular expression="," ("정규식")) -> (before substring=w348:string, after substring=w347:string)  [unwired: 1 in, 2 out]
                  n276 = call <vilib>:"GET.vi"("url"=w337) -> ("body"=w336:string, "error out"=w335:errorcluster)  [unwired: 11 in, 2 out]
                  n277 = Match Pattern "Clearance Delivery~Ground"(string=w336, regular expression="<!" ("문자열")) -> (after substring=w385:string)  [unwired: 1 in, 3 out]
                  n278 = Match Pattern "Clearance Delivery~Ground"(string=w385, regular expression=" html>" ("정규식")) -> (before substring=w382:string)  [unwired: 1 in, 3 out]
                  n279 = Equal?(x=w382, y="DOCTYPE") -> (x = y?=w342:bool)
                  n280 = case shown="거짓" w342 {
                    tunnel: w336 -> [w628 _]
                    frame False {
                      w622 = "\r"
                      # "x-offlinedata.pbfs"
                      n281 = local read "Destination"() -> (w624:string)
                      n282 = local read "departure"() -> (w627:string)
                      n283 = local read "Distance"() -> (w621:string)
                      n284 = To Upper Case(1:w624) -> (0:w625:string)
                      n285 = To Upper Case(1:w627) -> (0:w626:string)
                      n286 = Concatenate Strings(w626, w625, ":", w628, w622, "Distance" ("문자열"), w622, w621, "\r", "end", "\r") -> (w629:string)
                      n287 = call <vilib>:"Application Directory.vi"() -> ("Application Directory"=w616:path)
                      n288 = Build Array(w629) -> (w632:string[])
                      n289 = Path To String(path=w616) -> (string=w614:string)
                      n290 = Concatenate Strings(w614, "\\data\\x-offlinedata.pbfs" ("문자열")) -> (w615:string)
                      n291 = String To Path(string=w615) -> (path=w613:path)
                      n292 = call-poly <vilib>:"Write To Spreadsheet File.vi"("delimiter (\\t)"="\\n" ("delimiter (\\t)"), "transpose? (no:F)"=FALSE, "append to file? (new file:F)"=TRUE, "1D data"=w632, "file path (dialog if empty)"=w613) -> ()  [unwired: 3 in, 1 out]
                    }
                    frame True {
                    }
                  }
                  n293 = case shown="거짓" w340 {
                    tunnel: w341 -> [w602 _]
                    frame False {
                      w600 = "\r"
                      n294 = local read "Destination"() -> (w603:string)
                      n295 = local read "Distance"() -> (w599:string)
                      n296 = local read "departure"() -> (w605:string)
                      n297 = To Upper Case(1:w603) -> (0:w604:string)
                      n298 = To Upper Case(1:w605) -> (0:w606:string)
                      n299 = Concatenate Strings(w606, w604, ":", w600, w602, w600, "\tDistance", w600, w599, "\r", "end", "\r") -> (w607:string)
                      n300 = call <vilib>:"Application Directory.vi"() -> ("Application Directory"=w594:path)
                      n301 = Path To String(path=w594) -> (string=w592:string)
                      n302 = Build Array(w607) -> (w610:string[])
                      n303 = Concatenate Strings(w592, "\\data\\f-offlinedata.pbfs" ("문자열")) -> (w593:string)
                      n304 = String To Path(string=w593) -> (path=w591:path)
                      n305 = call-poly <vilib>:"Write To Spreadsheet File.vi"("delimiter (\\t)"="\\n" ("delimiter (\\t)"), "transpose? (no:F)"=FALSE, "append to file? (new file:F)"=TRUE, "1D data"=w610, "file path (dialog if empty)"=w591) -> ()  [unwired: 3 in, 1 out]
                    }
                    frame True {
                    }
                  }
                  n306 = Concatenate Strings(w348, w347) -> (w350:string)
                  n307 = Decimal String To Number(string=w350) -> (number=w352:i32)  [unwired: 2 in, 1 out]
                  n308 = Multiply(x=w352, y=1.85) -> (x*y=w343:dbl)
                  n309 = disable-structure shown="비활성화" {
                    disable-tunnel: w343 -> [w587 _]
                    frame Disabled {
                      n310 = Divide(x=w587, y=0.1041428571428571) -> (x/y=w588:dbl)
                      n311 = Multiply(x=w588, y=0.1) -> (x*y=w586:dbl)
                      n312 = Add(x=w588, y=w586) -> (x+y=w585:dbl)
                      n313 = Multiply(x=w585, y=2.204623) -> (x*y=w583:dbl)
                      n314 = To Long Integer(number=w583) -> ()  [unwired: 1 out]
                    }
                    frame Enabled {
                    }
                  }
                  n315 = call <vilib>:"Clear Errors.vi"("error in (no error)"=w335, "specific error code to clear (0: all)"=0) -> ()  [unwired: 4 in, 2 out]
                  n316 = Divide(x=w343, y=850.0) -> (x/y=w344:dbl)
                  n317 = case shown="거짓" w342 {
                    tunnel: w336 -> [w645 _]
                    frame False {
                      "x fmc 플랜" <- w645
                    }
                    frame True {
                      n318 = local write "x fmc 플랜"("찾을수 없습니다.") -> ()
                    }
                  }
                  n319 = case shown="참" w340 {
                    tunnel: w341 -> [w647 _]
                    frame False {
                      "fms" <- w647
                    }
                    frame True {
                      n320 = local write "FMS 플랜"("찾을수 없습니다.") -> ()
                    }
                  }
                  n321 = Number To Decimal String(number=w344) -> (decimal integer string=w369:string)  [unwired: 1 in]
                  n322 = Concatenate Strings(w369, "시간") -> ()  [unwired: 1 out]
                  n323 = Less Or Equal?(x=w344, y=0.5) -> (x <= y?=w346:bool)
                  n324 = case shown="거짓" w346 {
                    tunnel: w344 -> [w636 w637]
                    frame False {
                      n325 = Round To Nearest(number=w636) -> (nearest integer value=→"time/시간":dbl)
                    }
                    frame True {
                      n326 = local write "time/시간"(w637) -> ()
                    }
                  }
                  "FMS 플랜" <- w314
                }
              }
              frame 59 {
                n327 = while {
                  stop <- FALSE stop-if-true
                  w662 = "Distance" ("정규식")
                  w699 = T3 1 items=["사용자 홈"=0, "사용자 데스크탑"=1, "사용자 문서"=2, "사용자 어플리케이션 데이터"=3, "사용자 환경"=4, "사용자 임시"=5, "퍼블릭 문서"=6, "퍼블릭 어플리케이션 데이터"=7, "퍼블릭 환경"=8, "퍼블릭 캐시"=13, "시스템 코어 라이브러리"=9, "시스템 설치된 라이브러리"=10, "어플리케이션 파일"=11, "부팅 볼륨 루트"=12] ("system directory type")
                  w713 = T3 1 items=["사용자 홈"=0, "사용자 데스크탑"=1, "사용자 문서"=2, "사용자 어플리케이션 데이터"=3, "사용자 환경"=4, "사용자 임시"=5, "퍼블릭 문서"=6, "퍼블릭 어플리케이션 데이터"=7, "퍼블릭 환경"=8, "퍼블릭 캐시"=13, "시스템 코어 라이브러리"=9, "시스템 설치된 라이브러리"=10, "어플리케이션 파일"=11, "부팅 볼륨 루트"=12] ("system directory type")
                  n328 = local read "Destination"() -> (w693:string)
                  n329 = local read "departure"() -> (w695:string)
                  n330 = call <vilib>:"Get System Directory.vi"("system directory type"=w699) -> ("system directory"=w698:path)  [unwired: 10 in]
                  n331 = call <vilib>:"Get System Directory.vi"("system directory type"=w713) -> ("system directory"=w714:path)  [unwired: 10 in]
                  n332 = To Upper Case(1:w693) -> (0:w692:string)
                  n333 = Build Path(base path=w698, name or relative path="f-offlinedata.pbfs" ("이름 또는 상대 경로")) -> (appended path=w701:path)
                  n334 = To Upper Case(1:w695) -> (0:w694:string)
                  n335 = Build Path(base path=w714, name or relative path="x-offlinedata.pbfs" ("이름 또는 상대 경로")) -> (appended path=w711:path)
                  n336 = Concatenate Strings(w694, w692, ":") -> (w689:string)
                  n337 = Read from Text File(file (use dialog)=w701) -> (refnum out=w702:refnum<file>, text=w687:string, error out=w703:errorcluster)  [unwired: 3 in, 1 out]
                  n338 = Read from Text File(file (use dialog)=w711) -> (refnum out=w710:refnum<file>, text=w663:string, error out=w709:errorcluster)  [unwired: 3 in, 1 out]
                  n339 = Close File(refnum=w702, error in=w703) -> ()  [unwired: 2 out]
                  n340 = Close File(refnum=w710, error in=w709) -> ()  [unwired: 2 out]
                  n341 = Match Pattern(string=w663, regular expression=w689) -> (after substring=w691:string)  [unwired: 1 in, 3 out]
                  n342 = Match Pattern(string=w687, regular expression=w689) -> (after substring=w696:string)  [unwired: 1 in, 3 out]
                  n343 = Match Pattern(string=w696, regular expression="Distance") -> (before substring=w697:string)  [unwired: 1 in, 3 out]
                  n344 = Match Pattern(string=w691, regular expression=w662) -> (before substring=w690:string)  [unwired: 1 in, 3 out]
                  n345 = Match Pattern(string=w663, regular expression=w662) -> (after substring=w686:string)  [unwired: 1 in, 3 out]
                  n346 = Match Pattern(string=w686, regular expression="end" ("정규식")) -> (before substring=w676:string)  [unwired: 1 in, 3 out]
                  n347 = Equal?(x=w690, y="") -> (x = y?=w708:bool)
                  n348 = call <vilib>:"Trim Whitespace.vi"("string"=w676) -> ("trimmed string"=w682:string)  [unwired: 1 in]
                  n349 = Match Pattern "time/fuel"(string=w682, regular expression="nm" ("정규식")) -> (before substring=w678:string)  [unwired: 1 in, 3 out]
                  n350 = Match Pattern(string=w678, regular expression="," ("정규식")) -> (before substring=w680:string, after substring=w681:string)  [unwired: 1 in, 2 out]
                  n351 = Concatenate Strings(w680, w681) -> (w679:string)
                  n352 = Decimal String To Number(string=w679) -> (number=w667:i32)  [unwired: 2 in, 1 out]
                  n353 = Multiply(x=w667, y=1.85) -> (x*y=w666:dbl)
                  n354 = Divide(x=w666, y=850.0) -> (x/y=w664:dbl)
                  n355 = Equal?(x=w697, y="") -> (x = y?=w705:bool)
                  n356 = case shown="거짓" w705 {
                    tunnel: w697 -> [w716 _]
                    frame False {
                      n357 = local write "FMS 플랜"(w716) -> ()
                    }
                    frame True {
                      n358 = local write "x fmc 플랜"("오프라인  데이터에 없습니다. !" ("메시지")) -> ()
                    }
                  }
                  n359 = Divide(x=w666, y=0.1041428571428571) -> (x/y=w670:dbl)
                  n360 = Multiply(x=w670, y=0.1) -> (x*y=w671:dbl)
                  n361 = Add(x=w670, y=w671) -> (x+y=w672:dbl)
                  n362 = Multiply(x=w672, y=2.204623) -> (x*y=w674:dbl)
                  n363 = To Long Integer(number=w674) -> (32bit integer=w665:i32)
                  n364 = case shown="거짓" w708 {
                    tunnel: w690 -> [w722 _]
                    tunnel: w665 -> [_ _]
                    tunnel: w664 -> [w718 _]
                    tunnel: w664 -> [w719 _]
                    frame False {
                      n365 = Less Or Equal?(x=w719, y=0.5) -> (x <= y?=w721:bool)
                      n366 = local write "x fmc 플랜"(w722) -> ()
                      n367 = case shown="거짓" w721 {
                        tunnel: w718 -> [w723 w725]
                        frame False {
                          n368 = Round To Nearest(number=w723) -> (nearest integer value=w724:dbl)
                          n369 = local write "time/시간"(w724) -> ()
                        }
                        frame True {
                          n370 = local write "time/시간"(w725) -> ()
                        }
                      }
                    }
                    frame True {
                      n371 = local write "x fmc 플랜"("오프라인  데이터에 없습니다. !" ("메시지")) -> ()
                    }
                  }
                }
              }
            }
          }
        }
        n372 = local read "x fmc 플랜"() -> (w232:string)
        n373 = local read "x fmc 플랜"() -> (w239:string)
        n374 = local read "FMS 플랜"() -> (w227:string)
        n375 = local read "FMS 플랜"() -> (w237:string)
        n376 = local read "x fmc 플랜"() -> (w214:string)
        n377 = local read "FMS 플랜"() -> (w210:string)
        n378 = Equal?(x=w232, y="") -> (x = y?=w234:bool)
        n379 = Equal?(x=w239, y="찾을수 없습니다.") -> (x = y?=w240:bool)
        n380 = Equal?(x=w227, y="") -> (x = y?=w233:bool)
        n381 = Equal?(x=w237, y="찾을수 없습니다.") -> (x = y?=w241:bool)
        n382 = disable-structure shown="비활성화" {
          frame Disabled {
            w730 = T3 3 items=["사용자 홈"=0, "사용자 데스크탑"=1, "사용자 문서"=2, "사용자 어플리케이션 데이터"=3, "사용자 환경"=4, "사용자 임시"=5, "퍼블릭 문서"=6, "퍼블릭 어플리케이션 데이터"=7, "퍼블릭 환경"=8, "퍼블릭 캐시"=13, "시스템 코어 라이브러리"=9, "시스템 설치된 라이브러리"=10, "어플리케이션 파일"=11, "부팅 볼륨 루트"=12] ("system directory type")
            n383 = call <vilib>:"Get System Directory.vi"("create directory if not found? (F)"=TRUE, "system directory type"=w730) -> ("system directory"=w731:path)  [unwired: 9 in]
            n384 = Build Path(base path=w731, name or relative path="number.pbfs" ("이름 또는 상대 경로")) -> (appended path=w736:path)
            n385 = Open/Create/Replace File(file path (use dialog)=w736, operation (0:open)=T1."open or create" ("동작(0:open)"), access (0:read/write)=enum16{"read/write", "read-only", "write-only"}."write-only" ("접근(0:읽기/쓰기)")) -> (refnum out=w739:refnum<file>, error out=w728:errorcluster)  [unwired: 3 in, 1 out]
            n386 = call <vilib>:"Clear Errors.vi"("error in (no error)"=w728) -> ("error out"=w727:errorcluster)  [unwired: 5 in, 1 out]
            n387 = Write to Text File(file (use dialog)=w739, text="1" ("텍스트"), error in=w727) -> (refnum out=w740:refnum<file>, error out=w741:errorcluster)  [unwired: 1 in, 1 out]
            n388 = call <vilib>:"Clear Errors.vi"("error in (no error)"=w741, "specific error code to clear (0: all)"=0) -> ("error out"=w742:errorcluster)  [unwired: 4 in, 1 out]
            n389 = Close File(refnum=w740, error in=w742) -> (error out=w733:errorcluster)  [unwired: 1 out]
            n390 = call <vilib>:"Clear Errors.vi"("error in (no error)"=w733, "specific error code to clear (0: all)"=0) -> ()  [unwired: 4 in, 2 out]
          }
          frame Enabled {
          }
        }
        n391 = Equal?(x=w214, y="오프라인  데이터에 없습니다. !") -> (x = y?=w212:bool)
        n392 = Equal?(x=w210, y="오프라인  데이터에 없습니다. !") -> (x = y?=w213:bool)
        n393 = Or(x=w233, y=w234) -> (x .or. y?=w226:bool)
        n394 = And(x=w241, y=w240) -> (x .and. y?=w229:bool)
        n395 = Or(x=w213, y=w212) -> (x .or. y?=w211:bool)
        n396 = for {
          N: 1 -> [_]
          n397 = call <vilib>:"Application Directory.vi"() -> ("Application Directory"=w245:path)
          n398 = Path To String(path=w245) -> (string=w247:string)
          n399 = Concatenate Strings(w247, "\\data\\location.pbfs" ("문자열")) -> (w246:string)
          n400 = String To Path(string=w246) -> (path=w243:path)
          n401 = call <vilib>:"Open Config Data.vi"("create file if necessary (T)"=TRUE, "configuration file path"=w243) -> ("error out"=w250:errorcluster, "refnum"=w251:T2)  [unwired: 7 in, 1 out]
          n402 = call-poly <vilib>:"Write Key.vi"("section"="count", "error in (no error)"=w250, "value"="1", "key"="location", "refnum"=w251) -> ("error out"=w253:errorcluster, "refnum out"=w252:T2)  [unwired: 4 in, 1 out]
          n403 = call <vilib>:"Close Config Data.vi"("error in (no error)"=w253, "write file if changed (T)"=TRUE, "refnum"=w252) -> ()  [unwired: 7 in, 2 out]
        }
        n404 = Compound Arithmetic op=OR(w229, w226, w211) -> (w228:bool)
        n405 = case shown="거짓" w228 {
          frame False {
            n406 = local read "x fmc 플랜"() -> (w744:string)
            n407 = case shown="참" "?" {
              tunnel: w744 -> [_ w770]
              frame False {
              }
              frame True {
                (unwired) TRUE ("create directory if not found? (F)")
                n408 = local read "Destination"() -> (w777:string)
                n409 = local read "departure"() -> (w778:string)
                n410 = To Upper Case(1:w778) -> (0:w769:string)
                n411 = To Upper Case(1:w777) -> (0:w776:string)
                n412 = Concatenate Strings(w769, w776, ".FPL" ("문자열")) -> (w781:string)
                n413 = Build Path(base path="저장 경로", name or relative path=w781) -> (appended path=w784:path)
                n414 = Open/Create/Replace File(file path (use dialog)=w784, operation (0:open)=T1."open or create" ("동작(0:open)"), access (0:read/write)=enum16{"read/write", "read-only", "write-only"}."read/write" ("접근(0:읽기/쓰기)")) -> (refnum out=w786:refnum<file>, error out=w785:errorcluster)  [unwired: 3 in, 1 out]
                n415 = Write to Text File(file (use dialog)=w786, text=w770, error in=w785) -> (refnum out=w773:refnum<file>, error out=w775:errorcluster)  [unwired: 1 in, 1 out]
                n416 = call <vilib>:"Clear Errors.vi"("error in (no error)"=w775, "specific error code to clear (0: all)"=0) -> ("error out"=w774:errorcluster)  [unwired: 4 in, 1 out]
                n417 = Close File(refnum=w773, error in=w774) -> (error out=w771:errorcluster)  [unwired: 1 out]
                n418 = call <vilib>:"Clear Errors.vi"("error in (no error)"=w771) -> ()  [unwired: 5 in, 2 out]
              }
            }
            n419 = local read "fms"() -> (w746:string)
            n420 = case shown="참" "?" {
              tunnel: w746 -> [_ w763]
              frame False {
              }
              frame True {
                n421 = local read "Destination"() -> (w760:string)
                n422 = local read "departure"() -> (w759:string)
                n423 = To Upper Case(1:w760) -> (0:w751:string)
                n424 = To Upper Case(1:w759) -> (0:w753:string)
                n425 = local read "저장 경로"() -> (w755:path)
                n426 = Concatenate Strings(w753, "-" ("문자열"), w751, "_" ("문자열"), "GPS" ("문자열"), ".FMS" ("문자열")) -> (w761:string)
                n427 = Build Path(base path=w755, name or relative path=w761) -> (appended path=w765:path)
                n428 = Open/Create/Replace File(file path (use dialog)=w765, operation (0:open)=T1."open or create" ("동작(0:open)"), access (0:read/write)=enum16{"read/write", "read-only", "write-only"}."read/write" ("접근(0:읽기/쓰기)")) -> (refnum out=w768:refnum<file>, error out=w767:errorcluster)  [unwired: 3 in, 1 out]
                n429 = Write to Text File(file (use dialog)=w768, text=w763, error in=w767) -> (refnum out=w766:refnum<file>, error out=w758:errorcluster)  [unwired: 1 in, 1 out]
                n430 = call <vilib>:"Clear Errors.vi"("error in (no error)"=w758, "specific error code to clear (0: all)"=0) -> ("error out"=w757:errorcluster)  [unwired: 4 in, 1 out]
                n431 = Close File(refnum=w766, error in=w757) -> (error out=w754:errorcluster)  [unwired: 1 out]
                n432 = call <vilib>:"Clear Errors.vi"("error in (no error)"=w754) -> ()  [unwired: 5 in, 2 out]
              }
            }
          }
          frame True {
          }
        }
        n433 = call <vilib>:"Application Directory.vi"() -> ("Application Directory"=w204:path)
        n434 = Path To String(path=w204) -> (string=w202:string)
        n435 = Wait Until Next ms Multiple(millisecond multiple=u32 1000 ("ms 배수")) -> ()  [unwired: 1 out]
        n436 = local read "저장 경로"() -> (w218:path)
        n437 = Concatenate Strings(w202, "\\data\\location.pbfs" ("문자열")) -> (w203:string)
        n438 = String To Path(string=w203) -> (path=w201:path)
        n439 = call <vilib>:"Open Config Data.vi"("create file if necessary (T)"=TRUE, "configuration file path"=w201) -> ("error out"=w224:errorcluster, "refnum"=w223:T2)  [unwired: 7 in, 1 out]
        n440 = call-poly <vilib>:"Write Key.vi"("section"="location", "error in (no error)"=w224, "value"=w218, "key"="location", "refnum"=w223) -> ("error out"=w221:errorcluster, "refnum out"=w222:T2)  [unwired: 4 in, 1 out]
        n441 = call <vilib>:"Close Config Data.vi"("error in (no error)"=w221, "write file if changed (T)"=TRUE, "refnum"=w222) -> ()  [unwired: 7 in, 2 out]
      }
      n442 = while {
        tunnel: w154 -> [w157]
        stop <- FALSE stop-if-true
        n443 = event shown="[1] \"ATC\": 마우스 다운" {
          selector: _ -> [_ _ _ _]
          dyn-events: _ -> [_ _ _ _]
          timeout: 10 -> [_ _ _ _]
          tunnel: w157 -> [_ w160 _ _]
          event Timeout {
            n444 = event-data() -> ()  [unwired: 1 in, 3 out]
          }
          event "ATC": Mouse Down {
            n445 = event-data() -> ()  [unwired: 1 in, 8 out]
            n446 = case shown="거짓" w160 {
              frame False {
                w170 = 128  # call and forget
                n447 = vi-ref "ATCcont.vi"() -> (w163:refnum<vi>)
                n448 = property class="VI"(reference=w163) -> (error out=w164:errorcluster, "Path"=w165:path)  [unwired: 1 in, 1 out]
                n449 = Open VI Reference(type specifier VI Refnum (for type only)=refnum<vi> refnum, vi path=w165, options=w170, error in (no error)=w164) -> (vi reference=w162:refnum<vi>, error out=w168:errorcluster)  [unwired: 2 in]
                n450 = call-by-ref "Start Asynchronous Call"(reference=w162, error in=w168) -> (reference out=w161:refnum<vi>, error out=w167:errorcluster)  [unwired: 12 in]
                n451 = Close Reference(reference=w161, error in (no error)=w167) -> (error out=w166:errorcluster)
                n452 = call <vilib>:"Simple Error Handler.vi"("error in (no error)"=w166) -> ()  [unwired: 4 in, 5 out]
              }
              frame True {
                w180 = 128  # call and forget
                n453 = vi-ref "ATCpilot.vi"() -> (w173:refnum<vi>)
                n454 = property class="VI"(reference=w173) -> (error out=w174:errorcluster, "Path"=w175:path)  [unwired: 1 in, 1 out]
                n455 = Open VI Reference(type specifier VI Refnum (for type only)=refnum<vi> refnum, vi path=w175, options=w180, error in (no error)=w174) -> (vi reference=w172:refnum<vi>, error out=w178:errorcluster)  [unwired: 2 in]
                n456 = call-by-ref "Start Asynchronous Call"(reference=w172, error in=w178) -> (reference out=w171:refnum<vi>, error out=w177:errorcluster)  [unwired: 12 in]
                n457 = Close Reference(reference=w171, error in (no error)=w177) -> (error out=w176:errorcluster)
                n458 = call <vilib>:"Simple Error Handler.vi"("error in (no error)"=w176) -> ()  [unwired: 4 in, 5 out]
              }
            }
          }
          event "도움말": Mouse Down {
            w190 = 128  # call and forget
            n459 = event-data() -> ()  [unwired: 1 in, 8 out]
            n460 = vi-ref "rpopup.vi"() -> (w183:refnum<vi>)
            n461 = property class="VI"(reference=w183) -> (error out=w184:errorcluster, "Path"=w185:path)  [unwired: 1 in, 1 out]
            n462 = Open VI Reference(type specifier VI Refnum (for type only)=refnum<vi> refnum, vi path=w185, options=w190, error in (no error)=w184) -> (vi reference=w182:refnum<vi>, error out=w188:errorcluster)  [unwired: 2 in]
            n463 = call-by-ref "Start Asynchronous Call"(reference=w182, error in=w188) -> (reference out=w181:refnum<vi>, error out=w187:errorcluster)  [unwired: 12 in]
            n464 = Close Reference(reference=w181, error in (no error)=w187) -> (error out=w186:errorcluster)
            n465 = call <vilib>:"Simple Error Handler.vi"("error in (no error)"=w186) -> ()  [unwired: 4 in, 5 out]
          }
          event "피드백": Mouse Down {
            w200 = 128  # call and forget
            n466 = event-data() -> ()  [unwired: 1 in, 8 out]
            n467 = vi-ref "Feed.vi"() -> (w193:refnum<vi>)
            n468 = property class="VI"(reference=w193) -> (error out=w194:errorcluster, "Path"=w195:path)  [unwired: 1 in, 1 out]
            n469 = Open VI Reference(type specifier VI Refnum (for type only)=refnum<vi> refnum, vi path=w195, options=w200, error in (no error)=w194) -> (vi reference=w192:refnum<vi>, error out=w198:errorcluster)  [unwired: 2 in]
            n470 = call-by-ref "Start Asynchronous Call"(reference=w192, error in=w198) -> (reference out=w191:refnum<vi>, error out=w197:errorcluster)  [unwired: 12 in]
            n471 = Close Reference(reference=w191, error in (no error)=w197) -> (error out=w196:errorcluster)
            n472 = call <vilib>:"Simple Error Handler.vi"("error in (no error)"=w196) -> ()  [unwired: 4 in, 5 out]
          }
        }
      }
    }
  }
